vi "Test 3 Paths Cross in Future.vi"(8 "error in (no error)":errorcluster, 11 "Test Case In":refnum<class "Vector Test.lvclass">) -> (0 "error out":errorcluster, 3 "Test Case Out":refnum<class "Vector Test.lvclass">)   [LabVIEW 2021, in "Vector Test.lvclass"]
uses:
  Vector Test.lvclass
  C:/Program Files (x86)/National Instruments/LabVIEW 2021/vi.lib/Astemes/LUnit/Test Case.lvclass
  High Res Arithmetic/Rational Number.lvclass
  <vilib>/Astemes/LUnit/Test Case.lvclass/Test Case.ctl
  <vilib>/Astemes/LUnit/Append Fail Result.vi
  <vilib>/Astemes/LUnit/Append Pass Result.vi
  Vector/Vector.lvclass
  <vilib>/Astemes/LUnit/Test Case.lvclass
panel:
  out "Coordinate":T1
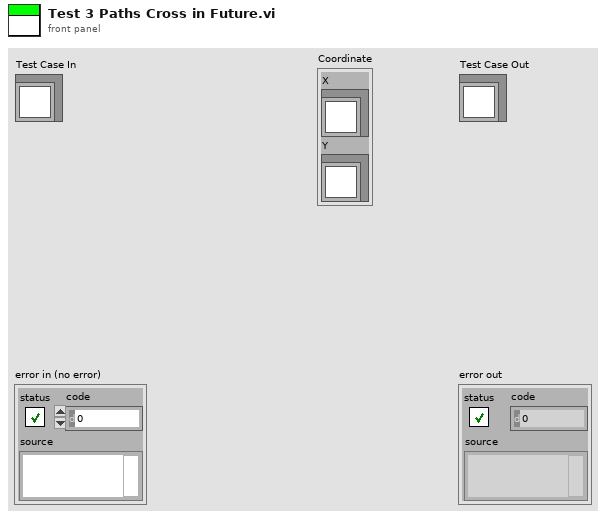
[diagram p1: front panel]
types:
  T1 = cluster{"X":refnum<class "Rational Number.lvclass">, "Y":refnum<class "Rational Number.lvclass">}
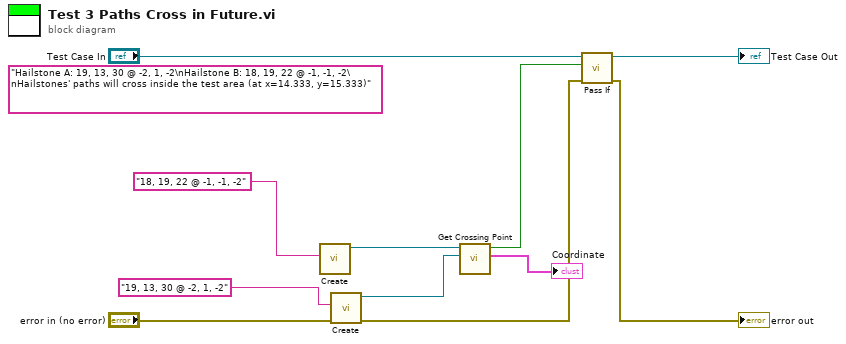
[diagram p0: block diagram]
diagram:
  (unwired) "Hailstone A: 19, 13, 30 @ -2, 1, -2\nHailstone B: 18, 19, 22 @ -1, -1, -2\nHailstones' paths will cross inside the test area (at x=14.333, y=15.333)" ("Input")
  n1 = call "Create.vi"("Input"="18, 19, 22 @ -1, -1, -2") -> ("Hailstone Out"=w4:refnum<class "Vector.lvclass">)  [unwired: 9 in, 1 out]
  n2 = call "Create.vi"("error in (no error)"="error in (no error)", "Input"="19, 13, 30 @ -2, 1, -2") -> ("error out"=w7:errorcluster, "Hailstone Out"=w3:refnum<class "Vector.lvclass">)  [unwired: 8 in]
  n3 = call "Get Crossing Point.vi"("Vector 2"=w3, "Vector in"=w4) -> ("Coordinate"=→"Coordinate":T1, "In Future?"=w2:bool)  [unwired: 8 in]
  n4 = call <vilib>:"Pass If.vi"("error in (no error)"=w7, "Pass?"=w2, "LUnit Test Case In"="Test Case In") -> ("error out"=→"error out":errorcluster, "LUnit Test Case Out"=→"Test Case Out":refnum<class "Vector Test.lvclass">)  [unwired: 7 in]
